vi "Digital Write Port Mega.vi"(0 "Arduino Resource":T1, 7 "Pin Values":bool[](array[boolean]), 11 "error in":errorcluster) -> (4 "Arduino Resource":T1, 15 "error out":errorcluster)   [LabVIEW 2009]
uses:
  <vilib>/LabVIEW Interface for Arduino/LabVIEW Interface for Arduino.lvlib
  <vilib>/LabVIEW Interface for Arduino/Type Defs/Board Type.ctl
  <vilib>/LabVIEW Interface for Arduino/Type Defs/Arduino Resource.ctl
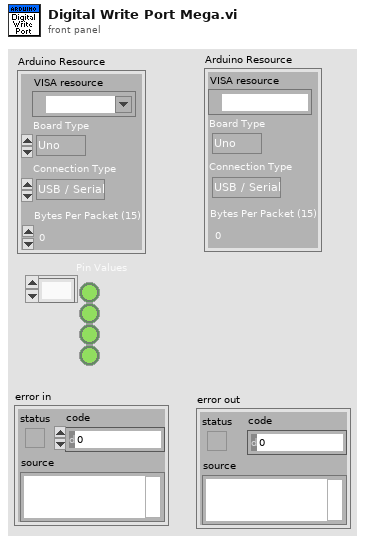
[diagram p1: front panel]
types:
  T1 = typedef "LabVIEW Interface for Arduino.lvlib/Arduino Resource.ctl" = cluster{"VISA resource":refnum<visa-resource-name>, "Board Type":T2, "Connection Type":enum8{"USB / Serial"}, "Bytes Per Packet (15)":u8}
  T2 = typedef "LabVIEW Interface for Arduino.lvlib/Board Type.ctl" = enum16{"Uno", "Dimuelanove w/Atmega 328", "Mega 2560"}
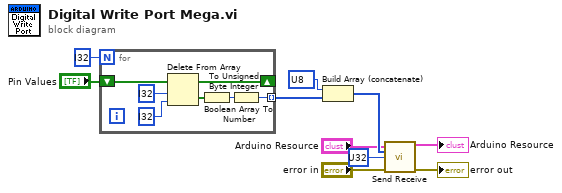
[diagram p0: block diagram]
diagram:
  n1 = for {
    N: i32 ? -> [_]
    shift-right: [w15] -> _
    shift-left: "Pin Values" -> [w17]
    tunnel: [w11] -> w2 mode=indexing
    n2 = Delete From Array(array=w17, length=i32 ?, index=i32 ?) -> (deleted portion=w14:bool[], array with subset deleted=w15:bool[])
    n3 = Boolean Array To Number(Boolean array=w14) -> (number=w16:u32)
    n4 = To Unsigned Byte Integer(number=w16) -> (unsigned 8bit integer=w11:u8)
  }
  n5 = Build Array (concatenate)(u8 ?, w2) -> (w10:u8[])
  n6 = call <vilib>:"Send Receive.vi"("Arduino Resource"="Arduino Resource", "Data"=w10, "Bytes To Read (0)"=u32 ?, "error in"="error in") -> ("Arduino Resource"=→"Arduino Resource":T1, "error out"=→"error out":errorcluster)  [unwired: 9 in, 1 out]
